vi "Read_spec_No_of_Characters.vi"(0 "Filename":path) -> (1 "character string":string, 2 "Error?":bool)   [LabVIEW 2010]
panel:
  out "error out":errorcluster
  out "Bytes to read":i32
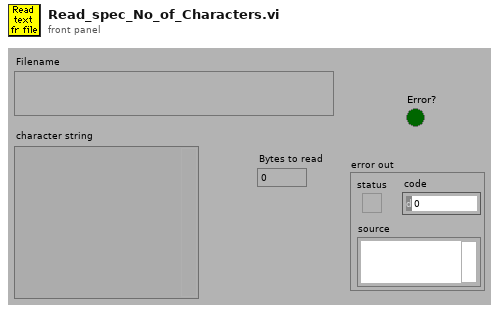
[diagram p1: front panel]
types:
  T1 = enum16{"read/write", "read-only", "write-only", "write-only (truncate)"}
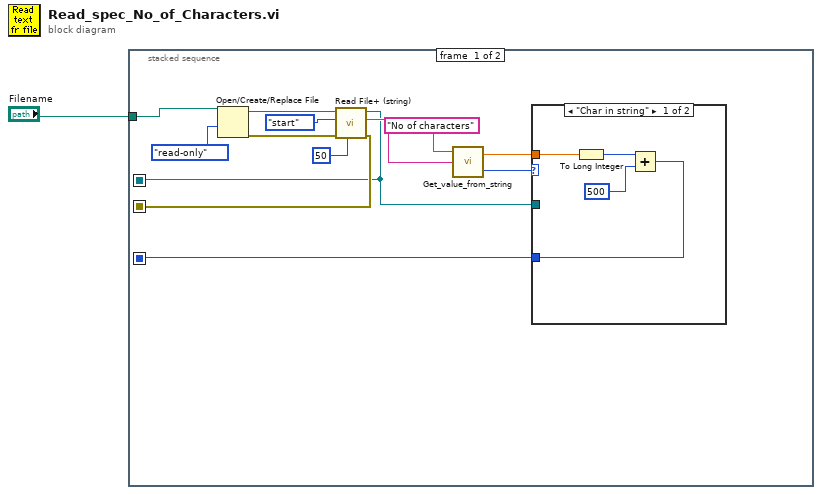
[diagram p0: block diagram]
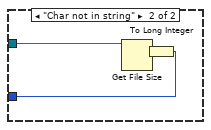
[diagram p2: hidden frame]
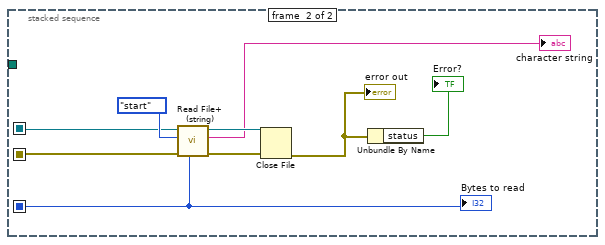
[diagram p3: hidden frame]
diagram:
  n1 = stacked-sequence {
    seq-local: [w12 _] -> [_ w27]
    seq-local: [w2 _] -> [_ w29]
    seq-local: [w4 _] -> [_ w28]
    tunnel: "Filename" -> [w9 _]
    frame #0 {
      n2 = Open/Create/Replace File(file path (use dialog)=w9, access (0:read/write)=T1."read-only" ("open mode (0)")) -> (refnum out=w6:refnum<file>, error out=w5:errorcluster)  [unwired: 1 in, 4 out]
      n3 = call <vilib>:"Read File+ (string).vi"("count"=50 ("number of characters (all:-1)"), "error in (no error)"=w5, "pos mode (rel. to current:2)"=enum16{"start", "end", "current"}."start", "refnum"=w6) -> ("error out"=w4:errorcluster, "string"=w3:string, "dup refnum"=w2:refnum<file>)  [unwired: 1 in, 4 out]
      n4 = call "Get_value_from_string.vi"("Input string"=w3, "Variable name"="No of characters") -> ("Status"=w13:enum16{"Char in string", "Char not in string"}, "Value"=w11:dbl)  [unwired: 1 in]
      n5 = case shown="\"Char in string\"" w13 {
        tunnel: [w16 w20] -> w12
        tunnel: w11 -> [w18 _]
        tunnel: w2 -> [_ w21]
        frame "Char in string" {
          n6 = To Long Integer(number=w18) -> (32bit integer=w17:i32)
          n7 = Add(x=w17, y=500) -> (x+y=w16:i32)
        }
        frame "Char not in string" {
          n8 = Get File Size(file=w21) -> (size (in bytes)=w19:i64)  [unwired: 1 in, 2 out]
          n9 = To Long Integer(number=w19) -> (32bit integer=w20:i32)
        }
      }
    }
    frame #1 {
      n10 = call <vilib>:"Read File+ (string).vi"("count"=w27, "error in (no error)"=w28, "pos mode (rel. to current:2)"=enum16{"start", "end", "current"}."start", "refnum"=w29) -> ("error out"=w25:errorcluster, "string"=→"character string":string, "dup refnum"=w26:refnum<file>)  [unwired: 1 in, 4 out]
      n11 = Close File(refnum=w26, error in=w25) -> (error out=w24:errorcluster)  [unwired: 1 out]
      "error out" <- w24
      n12 = Unbundle By Name(w24) -> ("status"=→"Error?":bool)
      "Bytes to read" <- w27
    }
  }
